vi "WriteWirelessEndpointAuths.vi"(8 "error in (no error)":errorcluster, 10 "SRP":T1, 11 "body":u8[](array[numeric])) -> (0 "error out":errorcluster)   [LabVIEW 2017, in "ServerComm.lvlib"]
uses:
  <vilib>/addons/InsightCM/Devices/Shared/Common/ServerComm/ServerComm.lvlib
  <vilib>/addons/InsightCM/SRP/controls/DVR_data.ctl
  <vilib>/addons/InsightCM/SRP/controls/data.ctl
  <vilib>/addons/InsightCM/MessageBus/Base/controls/EncryptedEndpointPasswords.ctl
  <vilib>/addons/InsightCM/Utilities/GlobalConfiguration/GlobalConfiguration.lvlib
  <vilib>/addons/InsightCM/SRP/SRP.lvlib
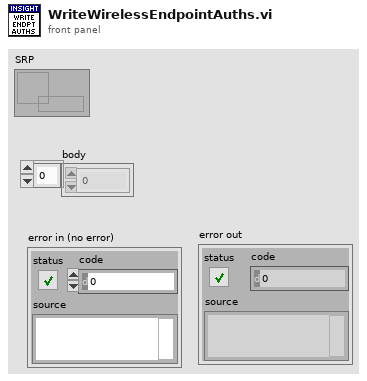
[diagram p1: front panel]
types:
  T1 = typedef "SRP.lvlib/DVR_data.ctl" = refnum<data-value>
  T2 = typedef "EncryptedEndpointPasswords.ctl" = cluster{"endpointAuthsIV":string, "WirelessEndpointAuths":string, "newPasswordsIV":string, "NewPasswordList":string}
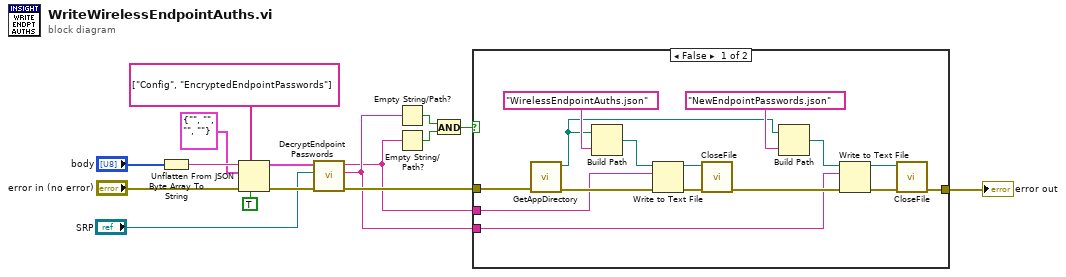
[diagram p0: block diagram]
diagram:
  n1 = Byte Array To String(unsigned byte array="body") -> (string=w12:string)
  n2 = Unflatten From JSON(path=string[] ["Config", "EncryptedEndpointPasswords"], JSON string=w12, type and defaults=T2 {"endpointAuthsIV"="", "WirelessEndpointAuths"="", "newPasswordsIV"="", "NewPasswordList"=""} ("EncryptedEndpointPasswords"), default null elements? (F)=TRUE, error in (no error)="error in (no error)") -> (value=w9:T2, error out=w10:errorcluster)  [unwired: 2 in]
  n3 = call <vilib>:"DecryptEndpointPasswords.vi"("error in (no error)"=w10, "srp"="SRP", "EncryptedEndpointPasswords"=w9) -> ("error out"=w7:errorcluster, "new password list"=w5:string, "wireless endpoint auths"=w4:string)  [unwired: 6 in]
  n4 = Empty String/Path?(string/path=w5) -> (empty?=w2:bool)
  n5 = Empty String/Path?(string/path=w4) -> (empty?=w1:bool)
  n6 = And(x=w2, y=w1) -> (x .and. y?=w3:bool)
  n7 = case shown="False" w3 {
    tunnel: w7 -> [w27 w32]
    tunnel: [w22 w32] -> w6
    tunnel: w4 -> [w19 _]
    tunnel: w5 -> [w17 _]
    frame False {
      n8 = call <vilib>:"GetAppDirectory.vi"("error in (no error)"=w27) -> ("error out"=w20:errorcluster, "application directory"=w21:path)  [unwired: 9 in]
      n9 = Build Path(base path=w21, name or relative path="WirelessEndpointAuths.json") -> (appended path=w30:path)
      n10 = Write to Text File(file (use dialog)=w30, text=w19, error in=w20) -> (refnum out=w29:refnum<file>, error out=w28:errorcluster)  [unwired: 1 in, 1 out]
      n11 = call <vilib>:"CloseFile.vi"("error in (no error)"=w28, "file reference"=w29) -> ("error out"=w18:errorcluster)  [unwired: 9 in]
      n12 = Build Path(base path=w21, name or relative path="NewEndpointPasswords.json") -> (appended path=w24:path)
      n13 = Write to Text File(file (use dialog)=w24, text=w17, error in=w18) -> (refnum out=w25:refnum<file>, error out=w26:errorcluster)  [unwired: 1 in, 1 out]
      n14 = call <vilib>:"CloseFile.vi"("error in (no error)"=w26, "file reference"=w25) -> ("error out"=w22:errorcluster)  [unwired: 9 in]
    }
    frame True {
    }
  }
  "error out" <- w6
